vi "Connect to URL.vi"(8 "Error In":errorcluster, 11 "URL":string) -> (0 "Error Out":errorcluster, 3 "Body":string)   [LabVIEW 2017]
uses:
  <vilib>/httpClient/LabVIEWHTTPClient.lvlib
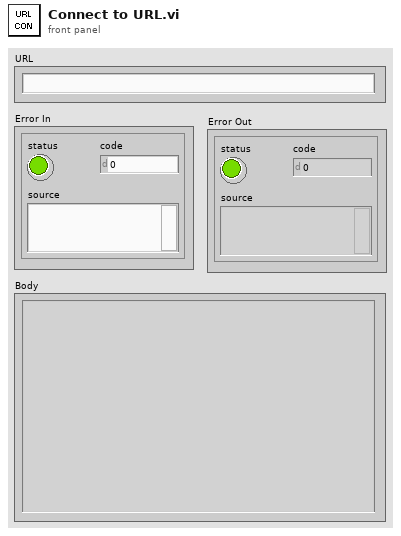
[diagram p1: front panel]
types:
  T1 = typedef "LabVIEWHTTPClient.lvlib/ClientHandle.ctl" = refnum<k1>
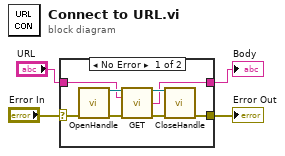
[diagram p0: block diagram]
diagram:
  n1 = case shown="No Error" "Error In" {
    selector: "Error In" -> [w7 w13]
    tunnel: "URL" -> [w8 _]
    tunnel: [w6 w13] -> w2
    tunnel: [w5 _] -> w1
    frame No Error {
      n2 = call <vilib>:"OpenHandle.vi"("error in (no error)"=w7) -> ("client handle out"=w12:T1, "error out"=w11:errorcluster)  [unwired: 13 in]
      n3 = call <vilib>:"GET.vi"("client handle"=w12, "url"=w8, "error in (no error)"=w11) -> ("client handle out"=w10:T1, "body"=w5:string, "error out"=w9:errorcluster)  [unwired: 9 in, 1 out]
      n4 = call <vilib>:"CloseHandle.vi"("client handle"=w10, "error in (no error)"=w9) -> ("error out"=w6:errorcluster)  [unwired: 13 in]
    }
    frame Error {
    }
  }
  "Error Out" <- w2
  "Body" <- w1
